vi "saveFocusFile.vi"(3 "tile_n_xy":cluster{"tile_n_x":i32, "tile_n_y":i32}, 4 "micro_pos-xyz":T2, 5 "q_tiles_x":dbl, 6 "focus_data":T1) -> (1 "focus_filename":string)   [LabVIEW 2014]
uses:
  GLOBAL_VAR.vi
panel:
  in  "folder_path":string="D:\\Data\\raw data\\"
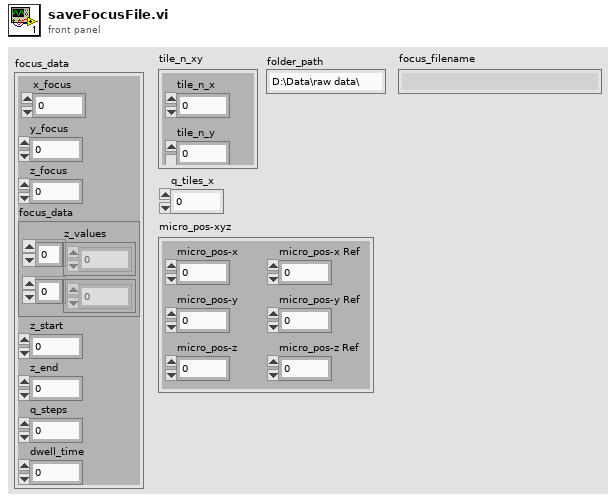
[diagram p1: front panel]
types:
  T1 = cluster{"x_focus":dbl, "y_focus":dbl, "z_focus":dbl, "focus_data":cluster{"z_values":dbl[], dbl[]}, "z_start":dbl, "z_end":dbl, "q_steps":i32, "dwell_time":dbl}
  T2 = cluster{"micro_pos-x":dbl, "micro_pos-y":dbl, "micro_pos-z":dbl, "micro_pos-x Ref":dbl, "micro_pos-y Ref":dbl, "micro_pos-z Ref":dbl}
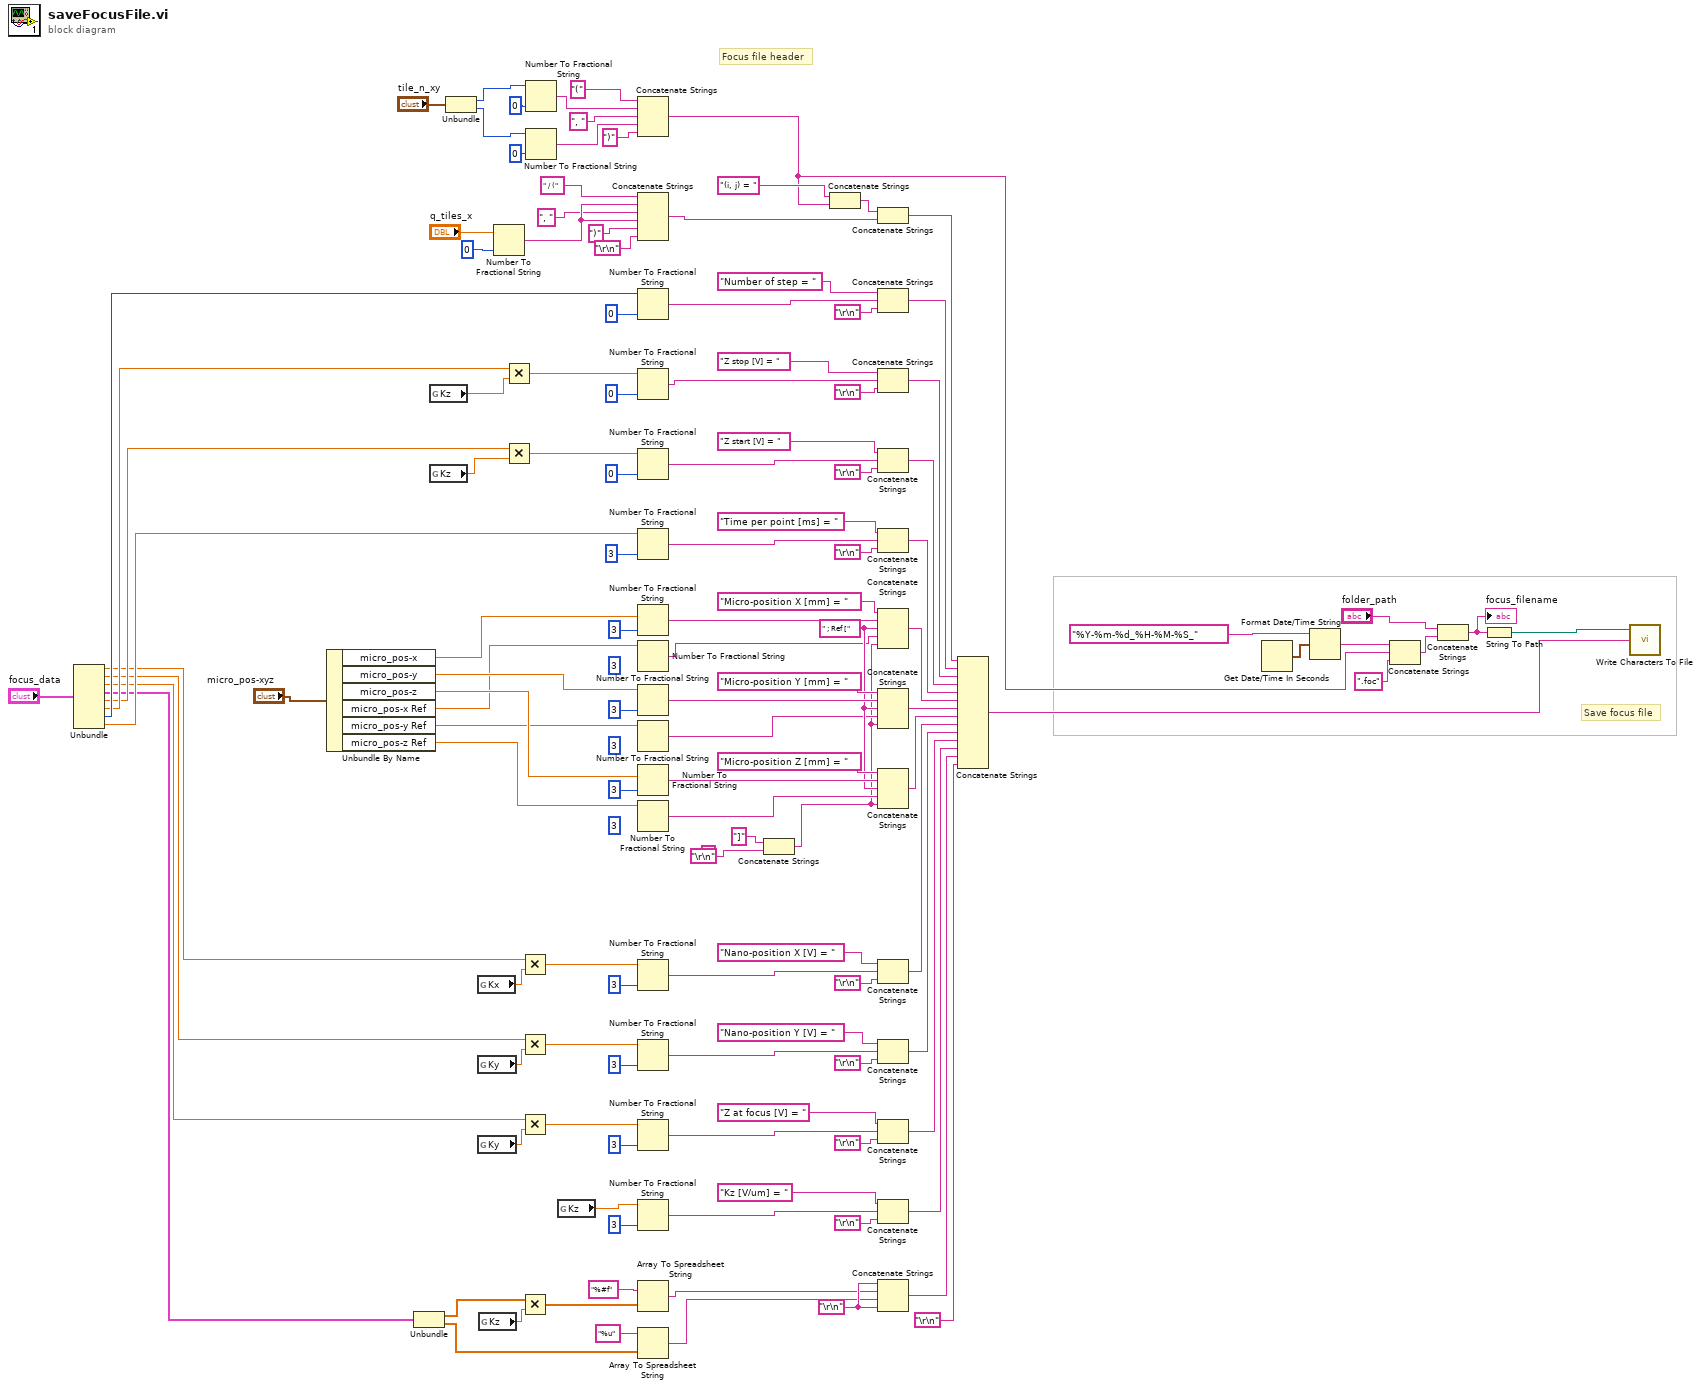
[diagram p0: block diagram]
diagram:
  (unwired) "" ("string")
  (unwired) i16 3 ("precision (6)")
  (unwired) i16 3 ("precision (6)")
  (unwired) i16 3 ("precision (6)")
  w10 = " ; Ref [" ("string")
  w116 = "\r\n"
  # "Save focus file"
  # "Focus file header"
  n1 = Unbundle("focus_data") -> ("x_focus"=w17:dbl, "y_focus"=w24:dbl, "z_focus"=w23:dbl, "focus_data"=w22:cluster{"z_values":dbl[], dbl[]}, "z_start"=w26:dbl, "z_end"=w27:dbl, "q_steps"=w28:i32, "dwell_time"=w25:dbl)
  n2 = Unbundle By Name("micro_pos-xyz") -> ("micro_pos-x"=w40:dbl, "micro_pos-y"=w39:dbl, "micro_pos-z"=w38:dbl, "micro_pos-x Ref"=w9:dbl, "micro_pos-y Ref"=w8:dbl, "micro_pos-z Ref"=w7:dbl)
  n3 = Unbundle(w22) -> ("z_values"=w126:dbl[], w127:dbl[])
  n4 = global read "GLOBAL_VAR.vi" "Kz"() -> (w36:dbl)
  n5 = global read "GLOBAL_VAR.vi" "Kz"() -> (w35:dbl)
  n6 = Unbundle("tile_n_xy") -> ("tile_n_x"=w47:i32, "tile_n_y"=w46:i32)
  n7 = global read "GLOBAL_VAR.vi" "Kx"() -> (w18:dbl)
  n8 = global read "GLOBAL_VAR.vi" "Ky"() -> (w31:dbl)
  n9 = global read "GLOBAL_VAR.vi" "Ky"() -> (w30:dbl)
  n10 = global read "GLOBAL_VAR.vi" "Kz"() -> (w19:dbl)
  n11 = Number To Fractional String(number="q_tiles_x", precision (6)=i16 0) -> (F-format string=w107:string)  [unwired: 2 in]
  n12 = Multiply(x=w27, y=w36) -> (x*y=w37:dbl)
  n13 = Multiply(x=w26, y=w35) -> (x*y=w34:dbl)
  n14 = Multiply(x=w17, y=w18) -> (x*y=w33:dbl)
  n15 = Multiply(x=w24, y=w31) -> (x*y=w32:dbl)
  n16 = Multiply(x=w23, y=w30) -> (x*y=w21:dbl)
  n17 = Multiply(x=w126, y=w19) -> (x*y=w20:dbl[])
  n18 = Number To Fractional String(number=w47, precision (6)=i16 0) -> (F-format string=w53:string)  [unwired: 2 in]
  n19 = Number To Fractional String(number=w46, precision (6)=i16 0) -> (F-format string=w55:string)  [unwired: 2 in]
  n20 = global read "GLOBAL_VAR.vi" "Kz"() -> (w12:dbl)
  n21 = Concatenate Strings("(", w53, ", ", w55, ")") -> (w50:string)
  n22 = Concatenate Strings(" / (", w107, ", ", w107, ")", "\r\n") -> (w109:string)
  n23 = Number To Fractional String(number=w28, precision (6)=i16 0) -> (F-format string=w69:string)  [unwired: 2 in]
  n24 = Number To Fractional String(number=w37, precision (6)=i16 0) -> (F-format string=w71:string)  [unwired: 2 in]
  n25 = Number To Fractional String(number=w34, precision (6)=i16 0) -> (F-format string=w73:string)  [unwired: 2 in]
  n26 = Number To Fractional String(number=w25, precision (6)=i16 3) -> (F-format string=w76:string)  [unwired: 2 in]
  n27 = Number To Fractional String(number=w40, precision (6)=i16 3) -> (F-format string=w79:string)  [unwired: 2 in]
  n28 = Number To Fractional String(number=w9) -> (F-format string=w6:string)  [unwired: 3 in]
  n29 = Number To Fractional String(number=w39, precision (6)=i16 3) -> (F-format string=w82:string)  [unwired: 2 in]
  n30 = Number To Fractional String(number=w8) -> (F-format string=w5:string)  [unwired: 3 in]
  n31 = Number To Fractional String(number=w38, precision (6)=i16 3) -> (F-format string=w44:string)  [unwired: 2 in]
  n32 = Number To Fractional String(number=w7) -> (F-format string=w4:string)  [unwired: 3 in]
  n33 = Number To Fractional String(number=w33, precision (6)=i16 3) -> (F-format string=w85:string)  [unwired: 2 in]
  n34 = Number To Fractional String(number=w32, precision (6)=i16 3) -> (F-format string=w90:string)  [unwired: 2 in]
  n35 = Number To Fractional String(number=w21, precision (6)=i16 3) -> (F-format string=w98:string)  [unwired: 2 in]
  n36 = Number To Fractional String(number=w12, precision (6)=i16 3) -> (F-format string=w15:string)  [unwired: 2 in]
  n37 = Array To Spreadsheet String(array=w20, 3:"%#f" ("format string")) -> (spreadsheet string=w115:string)  [unwired: 1 in]
  n38 = Array To Spreadsheet String(array=w127, 3:"%u" ("format string")) -> (spreadsheet string=w113:string)  [unwired: 1 in]
  n39 = Concatenate Strings("]" ("string"), "\r\n") -> (w1:string)
  n40 = Concatenate Strings("(i, j) = " ("string"), w50) -> (w111:string)
  n41 = Concatenate Strings(w111, w109) -> (w120:string)
  n42 = Concatenate Strings("Number of step = ", w69, "\r\n") -> (w121:string)
  n43 = Concatenate Strings("Z stop [V] = ", w71, "\r\n") -> (w124:string)
  n44 = Concatenate Strings("Z start [V] = ", w73, "\r\n") -> (w123:string)
  n45 = Concatenate Strings("Time per point [ms] = ", w76, "\r\n") -> (w122:string)
  n46 = Concatenate Strings("Micro-position X [mm] = ", w79, w10, w6, w1) -> (w92:string)
  n47 = Concatenate Strings("Micro-position Y [mm] = ", w82, w10, w5, w1) -> (w125:string)
  n48 = Concatenate Strings("Micro-position Z [mm] = ", w44, w10, w4, w1) -> (w41:string)
  n49 = Concatenate Strings("Nano-position X [V] = ", w85, "\r\n") -> (w42:string)
  n50 = Concatenate Strings("Nano-position Y [V] = ", w90, "\r\n") -> (w93:string)
  n51 = Concatenate Strings("Z at focus [V] = ", w98, "\r\n") -> (w100:string)
  n52 = Concatenate Strings("Kz [V/um] = ", w15, "\r\n") -> (w11:string)
  n53 = Concatenate Strings(w116, w115, w113, w116) -> (w103:string)
  n54 = Concatenate Strings(w120, w121, w124, w123, w122, w92, w125, w41, w42, w93, w100, w11, w103, "\r\n") -> (w102:string)
  n55 = Get Date/Time In Seconds() -> (seconds since 1Jan1904=w58:timestamp)
  n56 = Format Date/Time String(time format string (%c)="%Y-%m-%d_%H-%M-%S_", seconds (now)=w58) -> (date/time string=w59:string)  [unwired: 1 in]
  n57 = Concatenate Strings(w59, w50, ".foc") -> (w94:string)
  n58 = Concatenate Strings("folder_path", w94) -> (w118:string)
  "focus_filename" <- w118
  n59 = String To Path(string=w118) -> (path=w60:path)
  n60 = call <vilib>:"Write Characters To File.vi"("character string"=w102, "file path (dialog if empty)"=w60) -> ()  [unwired: 3 in, 1 out]
